vi "can开关切换.vi"(0 "输入切换ID":u8, 1 "输出切换ID":u8, 3 "CANID":u32 format="%x") -> (9 "成功？":bool)   [LabVIEW 2010]
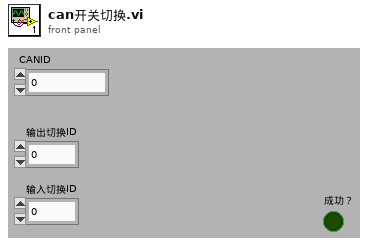
[diagram p1: front panel]
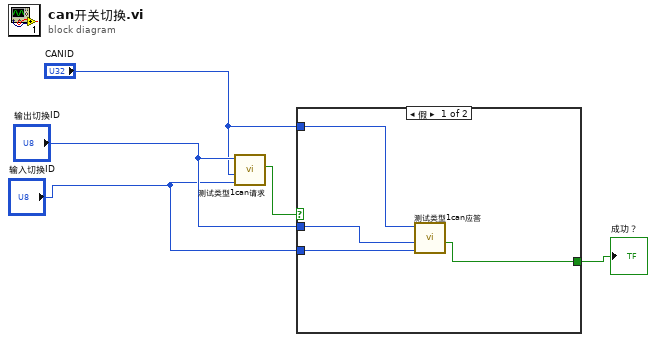
[diagram p0: block diagram]
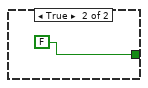
[diagram p2: hidden frame]
diagram:
  n1 = call "测试类型1can请求.vi"("输入切换ID"="输入切换ID", "CANID"="CANID", "输出切换ID"="输出切换ID") -> ("发送成功?"=w2:bool)  [unwired: 6 in]
  n2 = case shown="假" w2 {
    tunnel: [w9 FALSE] -> w5
    tunnel: "输出切换ID" -> [w8 _]
    tunnel: "输入切换ID" -> [w7 _]
    tunnel: "CANID" -> [w6 _]
    frame False {
      n3 = call "测试类型1can应答.vi"("输入切换ID"=w7, "输出切换ID"=w8, "匹配CANID"=w6) -> ("成功？"=w9:bool)  [unwired: 7 in]
    }
    frame True {
    }
  }
  "成功？" <- w5
